vi "Abort All.vi"(8 "error in (no error)":errorcluster, 11 "Sequencing Control in":refnum<class "Sequencing Control.lvclass">) -> (0 "error out":errorcluster, 3 "Sequencing Control out":refnum<class "Sequencing Control.lvclass">)   [LabVIEW 2020, in "VolatusSeqGUI.lvlib" / "Sequencing Control.lvclass"]
uses:
  Sequencing Control.lvclass
  Sequencing Control.lvclass/Sequencing Control.ctl
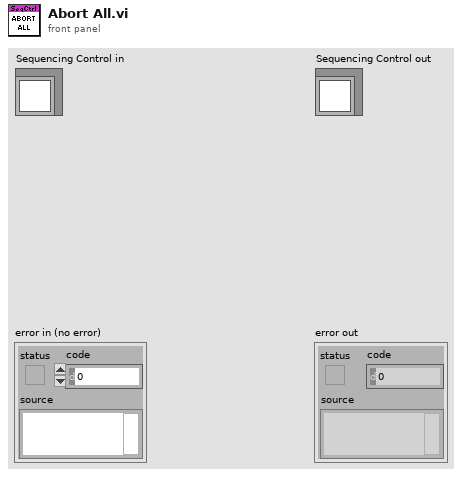
[diagram p1: front panel]
types:
  T1 = typedef "VolatusSeq.lvlib/Sequence Status JSON.ctl" = cluster{"name":string, "state":string, "running":bool, "abort":bool, "time":cluster{"seq":i64, "state":i64, "wall":i64}, "loaded":bool, "started":i64, "crc":u32, "color_bg":string, "error":errorcluster, "period":i64, "late":bool}
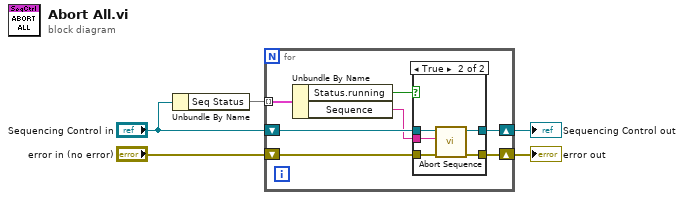
[diagram p0: block diagram]
diagram:
  n1 = Unbundle By Name("Sequencing Control in") -> ("Seq Status"=w1:map{string, T1})
  n2 = for {
    shift-right: [w11] -> w4
    shift-left: "error in (no error)" -> [w12]
    shift-right: [w10] -> w3
    shift-left: "Sequencing Control in" -> [w9]
    tunnel: w1 -> [w8] mode=indexing
    n3 = Unbundle By Name(w8) -> ("Status.running"=w6:bool, "Sequence"=w7:string)
    n4 = case shown="True" w6 {
      tunnel: w12 -> [w13 w19]
      tunnel: [w13 w18] -> w11
      tunnel: [w14 w17] -> w10
      tunnel: w9 -> [w14 w16]
      tunnel: w7 -> [_ w15]
      frame False {
      }
      frame True {
        n5 = call "Abort Sequence.vi"("error in (no error)"=w19, "Sequence Name"=w15, "Sequencing Control in"=w16) -> ("error out"=w18:errorcluster, "Sequencing Control out"=w17:refnum<class "Sequencing Control.lvclass">)  [unwired: 7 in]
      }
    }
  }
  "error out" <- w4
  "Sequencing Control out" <- w3
